vi "Blinking LED.vi"() -> ()   [LabVIEW 2014]
uses:
  libgpio_exp02.so
panel:
  out "Status 3":bool
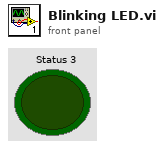
[diagram p1: front panel]
types:
  T1 = enum8{"INPUT", "OUTPUT", "PWM_OUTPUT", "GPIO_CLOCK", "SOFT_PWM_OUTPUT", "SOFT_TONE_OUTPUT", "PWM_TONE_OUTPUT"}
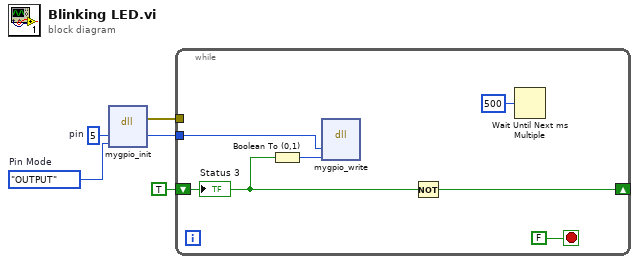
[diagram p0: block diagram]
diagram:
  w1 = T1."OUTPUT"  # Pin Mode
  w4 = u8 5  # pin
  n1 = dll-call lib="libgpio_exp02.so" fn="mygpio_init"("pin"=w4, "mode"=w1) -> (error out=w3:errorcluster, "pin"=w5:u8)  [unwired: 5 in, 1 out]
  n2 = while {
    tunnel: w3 -> [_]
    shift-right: [w7] -> _
    shift-left: TRUE -> [w10]
    tunnel: w5 -> [w6]
    stop <- FALSE stop-if-true
    n3 = Boolean To (0,1)(Boolean=w10) -> (0, 1=w11:i16)
    n4 = dll-call lib="libgpio_exp02.so" fn="mygpio_write"("pin"=w6, "state"=w11) -> ()  [unwired: 6 in, 2 out]
    n5 = Not(x=w10) -> (.not. x?=w7:bool)
    n6 = Wait Until Next ms Multiple(millisecond multiple=u32 500) -> ()  [unwired: 1 out]
    "Status 3" <- w10
  }
